vi "Initailize.vi"(8 "error in (no error)":errorcluster, 9 "zeromq.lvlib:ZeroMQ Context":refnum<class "zmq_context.lvclass">, 10 "Name":string, 11 "Channel Sub in":refnum<class "Channel Sub.lvclass">) -> (0 "error out":errorcluster, 3 "Channel Sub out":refnum<class "Channel Sub.lvclass">)   [LabVIEW 2018, in "Channel Sub.lvclass"]
uses:
  Channel Sub.lvclass
  <vilib>/addons/zeromq/zmq_context.lvclass
  Communication Channel/Communication Channel Folder/Communication Channel.lvclass
  Socket2/Socket2/Socket2.lvclass
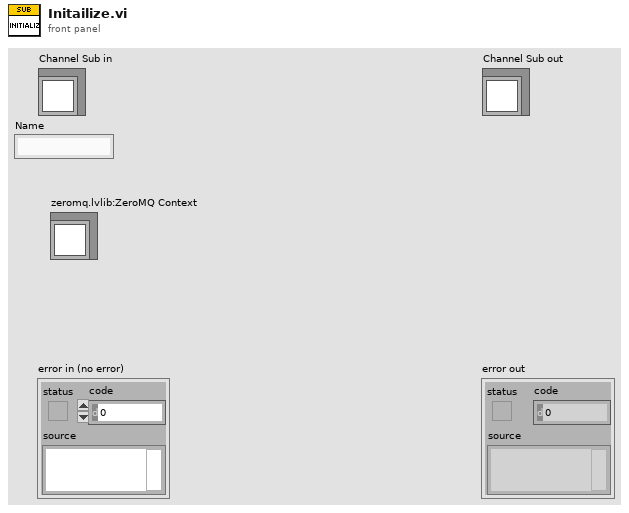
[diagram p1: front panel]
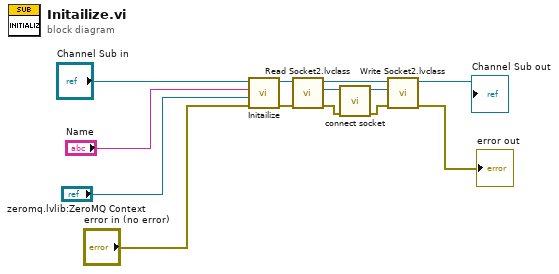
[diagram p0: block diagram]
diagram:
  n1 = call-parent "Initailize.vi"("error in (no error)"="error in (no error)", "zeromq.lvlib:ZeroMQ Context"="zeromq.lvlib:ZeroMQ Context", "Name"="Name", "Communication Channel in"="Channel Sub in") -> ("error out"=w8:errorcluster, "Communication Channel out"=w9:refnum<class "Channel Sub.lvclass">)  [unwired: 6 in]
  n2 = call-dynamic "Read Socket2.lvclass.vi"("error in (no error)"=w8, "Communication Channel in"=w9) -> ("error out"=w4:errorcluster, "Socket2.lvclass"=w6:refnum<class "Socket2.lvclass">, "Communication Channel out"=w7:refnum<class "Channel Sub.lvclass">)  [unwired: 7 in]
  n3 = call "connect socket.vi"("error in (no error)"=w4, "Socket in"=w6) -> ("error out"=w3:errorcluster, "Socket out"=w5:refnum<class "Socket2.lvclass">)  [unwired: 8 in]
  n4 = call-dynamic "Write Socket2.lvclass.vi"("error in (no error)"=w3, "Socket2.lvclass"=w5, "Communication Channel in"=w7) -> ("error out"=→"error out":errorcluster, "Communication Channel out"=→"Channel Sub out":refnum<class "Channel Sub.lvclass">)  [unwired: 7 in]
